vi "AK-LNI Remote Mode.vi"(7 "Kanalnummer (K0)":u8 max=99 step=1, 8 "Fehler (Eingang)":errorcluster, 10 "Remote":bool, 11 "VISA resource name":refnum<visa-resource-name>) -> (0 "Fehler (Ausgang)":errorcluster, 1 "ES (Error Status)":string, 3 "VISA resource name out":refnum<visa-resource-name>)   [LabVIEW 2015, in "Linearisierung v2.lvlib" / "Gasteiler.lvlib" / "AK Komm Gasteiler.lvlib"]
doc: "\"Remote\" = TRUE: schaltet in den Fernsteuer-Betrieb (Remote command mode).\n\"Remote\" = FALSE: kehrt in den LCD-Betrieb zurück (Manual command mode)."
uses:
  AK Komm Gasteiler.lvlib
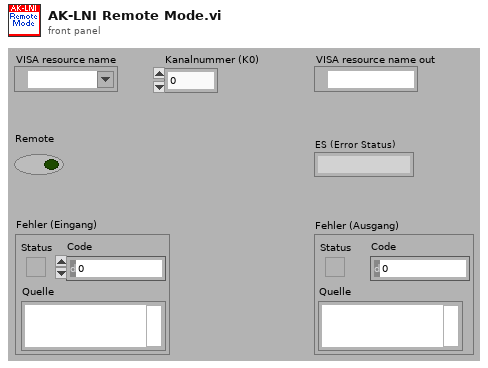
[diagram p1: front panel]
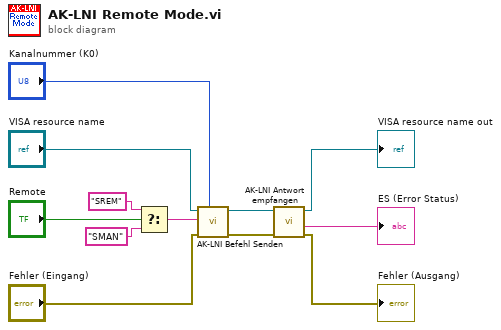
[diagram p0: block diagram]
diagram:
  n1 = Select(t="SREM" ("Befehl (2 Zeichen erf.)"), s="Remote", f="SMAN") -> (s? t:f=w2:string)
  n2 = call "AK-LNI Befehl Senden.vi"("Kanalnummer (K0)"="Kanalnummer (K0)", "Fehler (Eingang)"="Fehler (Eingang)", "Befehl (4 Zeichen)"=w2, "VISA resource name"="VISA resource name") -> ("Fehler (Ausgang)"=w6:errorcluster, "VISA resource name out"=w11:refnum<visa-resource-name>)  [unwired: 6 in]
  n3 = call "AK-LNI Antwort empfangen.vi"("Fehler (Eingang)"=w6, "VISA resource name"=w11) -> ("Fehler (Ausgang)"=→"Fehler (Ausgang)":errorcluster, "ES (Error Status)"=→"ES (Error Status)":string, "VISA resource name out"=→"VISA resource name out":refnum<visa-resource-name>)  [unwired: 4 in, 3 out]
